vi "Delay Error Message.vi"(2 "error in (no error)":errorcluster, 3 "Seconds since 1904":dbl) -> ()   [LabVIEW 2020]
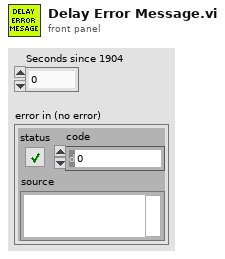
[diagram p1: front panel]
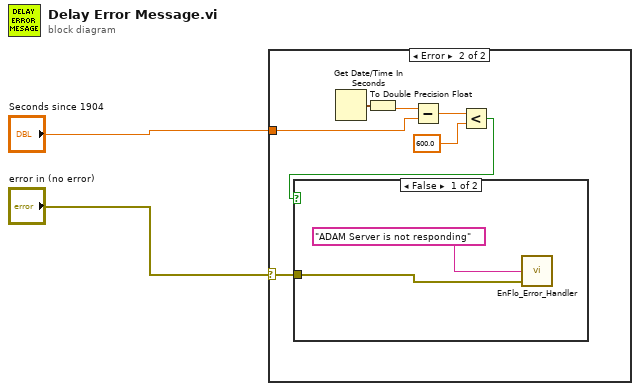
[diagram p0: block diagram]
diagram:
  n1 = case shown="Error" "error in (no error)" {
    selector: "error in (no error)" -> [_ w3]
    tunnel: "Seconds since 1904" -> [_ w5]
    frame No Error {
    }
    frame Error {
      n2 = Get Date/Time In Seconds() -> (seconds since 1Jan1904=w9:timestamp)
      n3 = To Double Precision Float(number=w9) -> (double precision float=w8:dbl)
      n4 = Subtract(x=w8, y=w5) -> (x-y=w7:dbl)
      n5 = Less?(x=w7, y=600.0) -> (x < y?=w4:bool)
      n6 = case shown="False" w4 {
        tunnel: w3 -> [w11 _]
        frame False {
          n7 = call "EnFlo_Error_Handler.vi"("error in (no error)"=w11, "Error Type"="ADAM Server is not responding") -> ()  [unwired: 1 in, 3 out]
        }
        frame True {
        }
      }
    }
  }
